vi "cargarDatoImagen.vi"(11 "IndiceAUltimoValor\nAgregadoEnLaTabla":i32=1) -> ()   [LabVIEW 2014]
uses:
  claseImagen/claseImagen.lvclass
panel:
  out "dataReading":T1
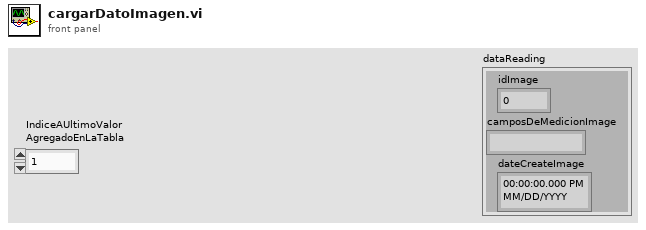
[diagram p1: front panel]
types:
  T1 = cluster{"idImage":dbl, "camposDeMedicionImage":string, "dateCreateImage":timestamp}
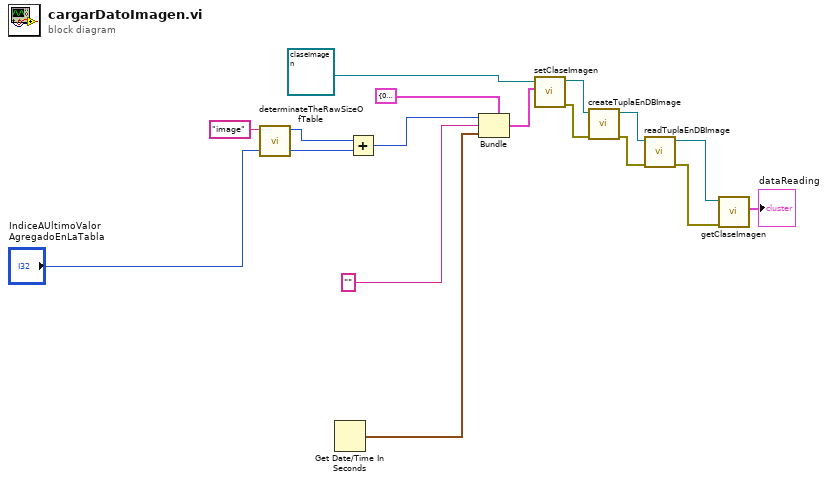
[diagram p0: block diagram]
diagram:
  n1 = call "determinateTheRawSizeOfTable.vi"("tableName"="image") -> ("sizeOfTableInNumberRaw"=w2:i32)  [unwired: 8 in, 1 out]
  n2 = Get Date/Time In Seconds() -> (seconds since 1Jan1904=w10:timestamp)
  n3 = Add(x=w2, y="IndiceAUltimoValor\nAgregadoEnLaTabla") -> (x+y=w11:i32)
  n4 = Bundle(cluster=T1 {"idImage"=0.0, "camposDeMedicionImage"="", "dateCreateImage"=timestamp(0 s since 1904-01-01)} ("ImageDataIn"), "idImage"=w11, "camposDeMedicionImage"="", "dateCreateImage"=w10) -> (w12:T1)
  n5 = call "setClaseImagen.vi"("ImageDataIn"=w12, "claseImagen in"=refnum<class "claseImagen.lvclass"> refnum ("claseImagen.lvclass")) -> ("error out"=w7:errorcluster, "claseImagen out"=w8:refnum<class "claseImagen.lvclass">)  [unwired: 8 in]
  n6 = call "createTuplaEnDBImage.vi"("claseImagen in"=w8, "error in"=w7) -> ("claseImagen out"=w6:refnum<class "claseImagen.lvclass">, "error out"=w5:errorcluster)  [unwired: 7 in]
  n7 = call "readTuplaEnDBImage.vi"("error in"=w5, "claseImagen in"=w6) -> ("error out"=w3:errorcluster, "claseImagen out"=w4:refnum<class "claseImagen.lvclass">)  [unwired: 8 in]
  n8 = call "getClaseImagen.vi"("error in"=w3, "claseImagen in"=w4) -> ("dataReading"=→"dataReading":T1)  [unwired: 7 in, 2 out]
